vi "Build Greater Equal 0 Compare Types.vi"   [LabVIEW 2021]
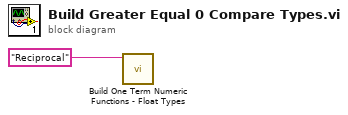
[diagram p0: block diagram]
diagram:
  n1 = call "Build One Term Numeric Functions - Float Types.vi"("Comparison Name"="Reciprocal") -> ()  [unwired: 11 in]
